vi "XIPIN_Object_Segmentation_3_00_a.vi"   [LabVIEW 2017]
doc: "The Xilinx Object Segmentation LogiCORE is used in conjunction with the Xilinx Image Characterization LogiCORE, to convert the statistical data provided into a list of objects that meet a user-defined set of object characteristics. This core provides an easy hardware-accelerated method for establishing up to 8 combinations of features. Each feature set is defined by upper and lower thresholds imposed on the statistical data obtained from the Image Characterization LogiCORE. The core further provides a mechanism for logically combining up to 4 of the feature sets selected above to extend the segmentation capabilities of the core. Up to 31 objects are supported by aggregating the neighboring image blocks that meet the characteristics of this user defined set of characteristics into a single object. The core is programmable through a comprehensive register interface.\n------------------------------------\n<b>Need License</b> : Yes\n<b>Interface</b> : AXI4-Stream AXI4-Lite"
uses:
  <vilib>/rvi/XilinxIP/XIPIN_XNode/niFpgaXIPIN.xnode
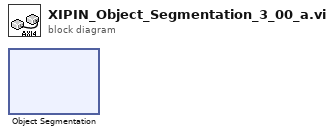
[diagram p0: block diagram]
diagram:
  n1 = xnode ("Object Segmentation")() -> ()
